vi "getStopMechanism.vi"(8 "error in (no error)":errorcluster, 11 "ITaskClassTemplate in":refnum<class "ITaskClassTemplate.lvclass">) -> (0 "error out":errorcluster, 2 "stopMechanism":refnum<class "ITaskStopMechanism.lvclass">, 3 "ITaskClassTemplate out":refnum<class "ITaskClassTemplate.lvclass">)   [LabVIEW 2023, in "ITaskClassTemplate.lvclass"]
doc: "Returns the stop mechanism type used by the task.\n_____________________________________\nTLC Daemon 1.0.0.6\nCopyright (c) 2026 Andrea Cadei"
uses:
  ITaskClassTemplate.lvclass
  ITaskClassTemplate.lvclass/ITaskClassTemplate.ctl
  BoolNotifierStopMech/BoolNotifierStopMechanism.lvclass
  BoolUserEventStopMech/BoolUserEventStopMechanism.lvclass
  MsgUserEventStopMech/MsgUserEventStopMechanism.lvclass
  ITaskStopMechanism/ITaskStopMechanism.lvclass
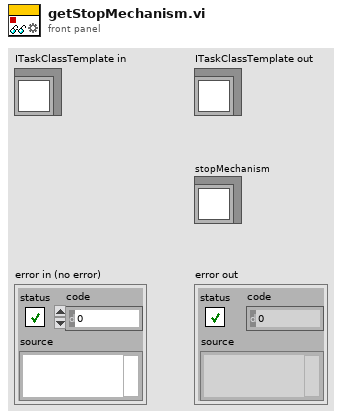
[diagram p1: front panel]
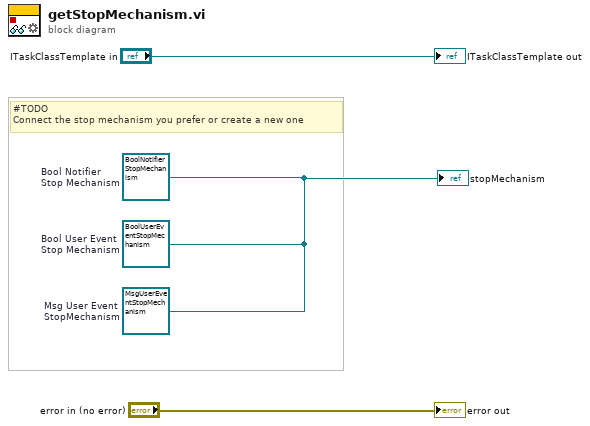
[diagram p0: block diagram]
diagram:
  w1 = refnum<class "MsgUserEventStopMechanism.lvclass"> refnum  # Msg User Event StopMechanism
  w1 = refnum<class "BoolUserEventStopMechanism.lvclass"> refnum  # Bool User Event Stop Mechanism
  w1 = refnum<class "BoolNotifierStopMechanism.lvclass"> refnum  # Bool Notifier  Stop Mechanism
  # "#TODO\nConnect the stop mechanism you prefer or create a new one"
  "error out" <- "error in (no error)"
  "ITaskClassTemplate out" <- "ITaskClassTemplate in"
  "stopMechanism" <- w1
